vi "slides.vi"() -> ()   [LabVIEW 2020]
uses:
  <instrlib>/_niInstr/Network/IPv4/UDP/Data Stream/v1/niInstr IPv4 UDP Data Stream v1.lvclass
  <instrlib>/_niInstr/Network/IPv4/UDP/Data Stream/v1/Read Data Stream.vi
  <instrlib>/_niInstr/Network/Ethernet/Utility/v1/FPGA/niInstr Ethernet Utilities FPGA v1.lvlib
  <instrlib>/_niInstr/Network/IPv4/FPGA/v1/niInstr IPv4 FPGA v1.lvlib
  <instrlib>/_niInstr/Network/IPv4/UDP/FPGA/v1/niInstr IPv4 UDP FPGA v1.lvlib
  Ethernet MAC - Custom/Ethernet MAC - Custom.lvclass
  <vilib>/rvi/DataTransferAndStorage/Container/XNode/niFpgaContainer.xnode
  <instrlib>/_niInstr/Network/IPv4/UDP/Data Stream/v1/Read End of Good Frame.vi
  <instrlib>/_niInstr/Network/IPv4/UDP/Data Stream/v1/Read End of Bad Frame.vi
  submodules/Market.Data.Common/fpga/my.network.data.stream.ctl
  <vilib>/rvi/FIFO/Fifo_Resource/niFpgaFifoEmulationRefIn.vi
  <instrlib>/_niInstr/Network/Types/v1/MAC Address.ctl
  <instrlib>/_niInstr/Network/Types/v1/niInstr Network Types v1.lvlib
  <instrlib>/_niInstr/Network/Types/v1/IPv4 Address.ctl
  submodules/Market.Data.Common/fpga/orderbook.command.type.ctl
  submodules/Market.Data.Common/fpga/fpganow.common.fpga.lvlib
  submodules/Market.Data.Common/fpga/orderbook.command.ctl
panel:
  out "remaining.qty":u32
  out "seconds":u64
  out "nanoseconds":u64
  out "Add":bool
  out "Edit":bool
  out "Remove":bool
  out "seq no":u32
  out "recv.time":u64
  out "parse.time":u64
  out "canceled.qty":u32
  out "executed.qty":u32
  out "price":u64
  out "symbol":u64
  out "quantity":u32
  out "orderId":u64
  out "side":u8
  out "type":T1
  in  "OrderBook.Command":T2={"type"=enum."AddOrder", "side"=0, "orderId "=0, "quantity"=0, "symbol"=0, "price"=0, "executed.qty"=0, "canceled.qty"=0, "remaining.qty"=0, "seconds"=0, "nanoseconds"=0, "Add"=FALSE, "Edit"=FALSE, "Remove"=FALSE, "seq no"=0, "recv.time"=0, "parse.time"=0}
  in  "Dest Port":u16=8000
  in  "IP Address":T3=[176, 197, 84, 255]
  in  "MAC Address":T4=[176, 197, 84, 255, 244, 135] format="%.0x"
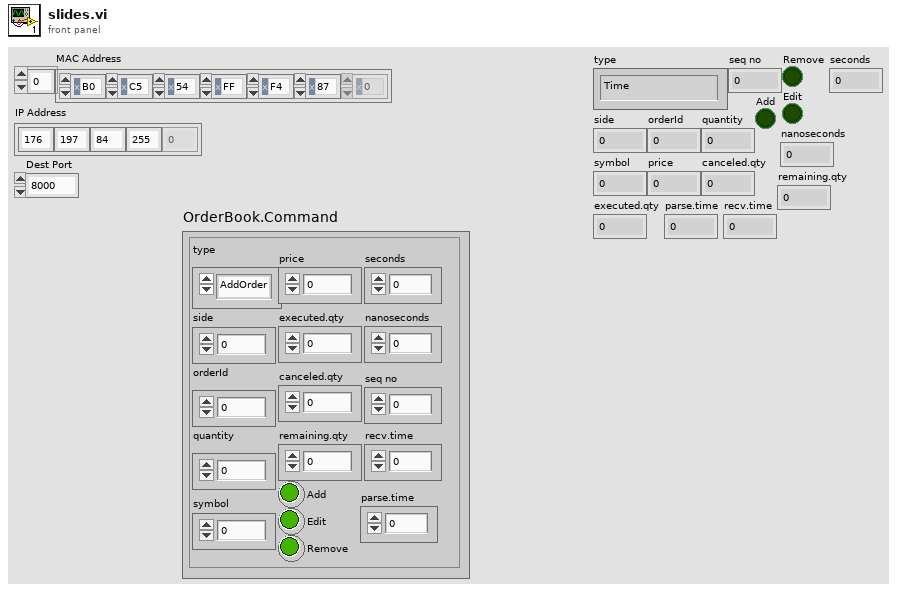
[diagram p1: front panel]
types:
  T1 = typedef "fpganow.common.fpga.lvlib/orderbook.command.type.ctl" = enum8{"Time", "AddOrder", "OrderExecuted", "OrderExecutedAtPrice", "ReduceSize", "ModifyOrder", "DeleteOrder", "Get.Everything", "Get.All.Orders", "Get.Top"}
  T2 = typedef "fpganow.common.fpga.lvlib/orderbook.command.ctl" = cluster{"type":T1, "side":u8, "orderId ":u64, "quantity":u32, "symbol":u64, "price":u64, "executed.qty":u32, "canceled.qty":u32, "remaining.qty":u32, "seconds":u64, "nanoseconds":u64, "Add":bool, "Edit":bool, "Remove":bool, "seq no":u32, "recv.time":u64, "parse.time":u64}
  T3 = typedef "niInstr Network Types v1.lvlib/IPv4 Address.ctl" = u8[]
  T4 = typedef "niInstr Network Types v1.lvlib/MAC Address.ctl" = u8[]
  T5 = typedef "my.network.data.stream.ctl" = cluster{"data":u8[], "data valid":bool, "byte enables":bool[], "eof.good":bool, "eof.bad":bool, "Timestamp":u64}
  T6 = typedef "niInstr Ethernet Utilities FPGA v1.lvlib/Network Data Stream.ctl" = cluster{"data":u8[], "data valid":bool, "byte enables":bool[]}
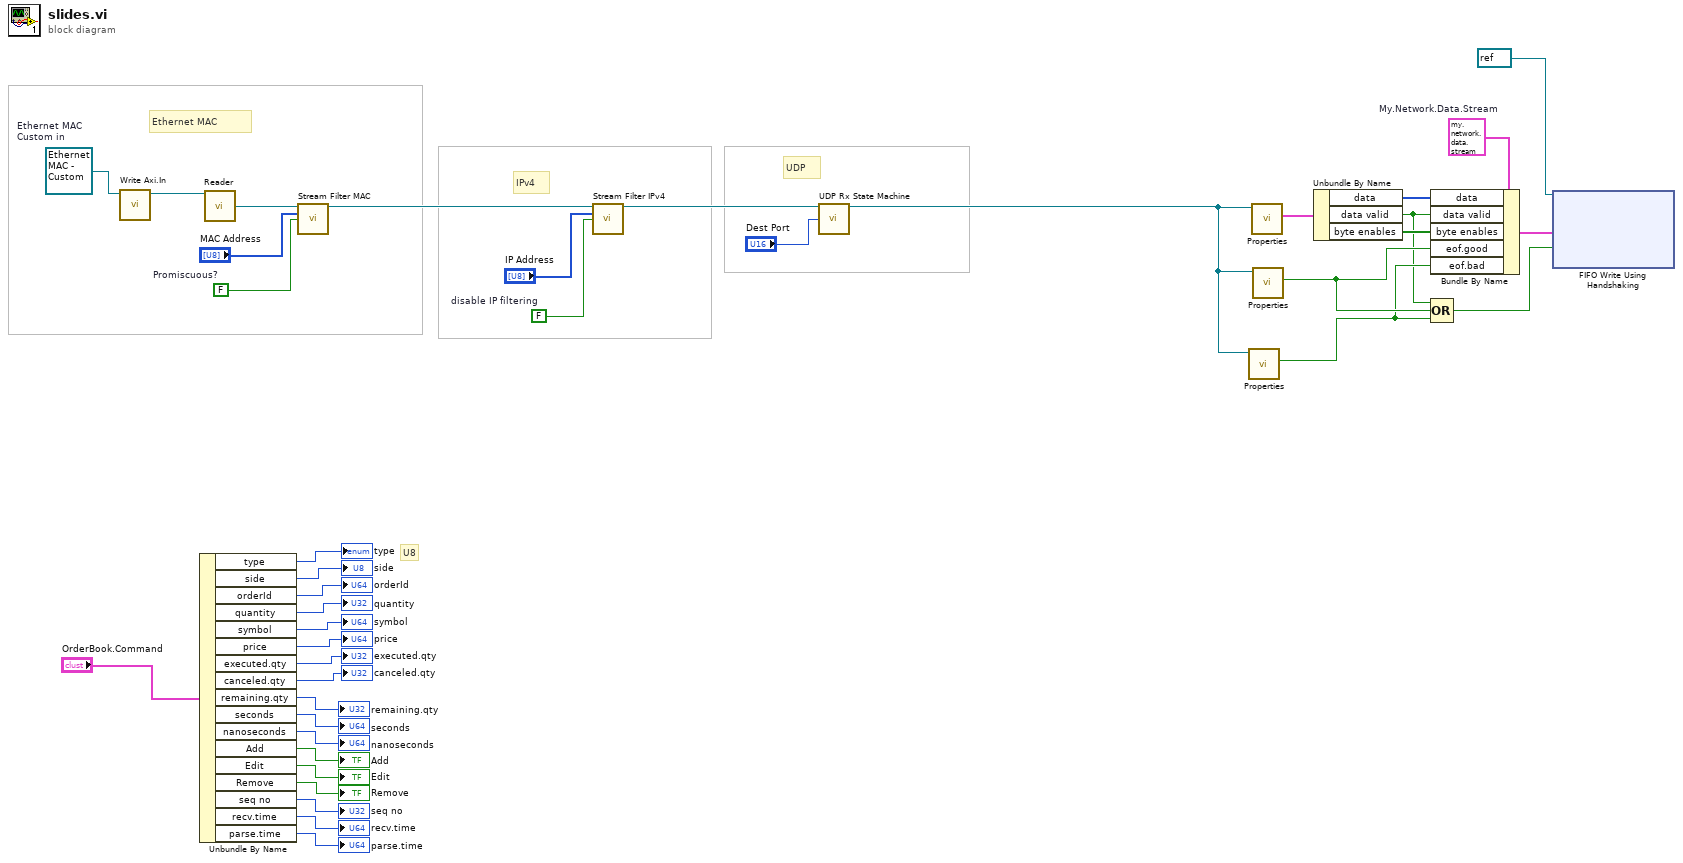
[diagram p0: block diagram]
diagram:
  w29 = T5 {"data"=[0, 0, 0, 0, 0, 0, 0, 0], "data valid"=FALSE, "byte enables"=[FALSE, FALSE, FALSE, FALSE, FALSE, FALSE, FALSE, FALSE], "eof.good"=FALSE, "eof.bad"=FALSE, "Timestamp"=0}  # My.Network.Data.Stream
  w31 = refnum<class "Ethernet MAC - Custom.lvclass"> refnum  # Ethernet MAC Custom in
  w36 = FALSE  # disable IP filtering
  w37 = FALSE  # Promiscuous?
  # "U8"
  # "UDP"
  # "IPv4"
  # "Ethernet MAC"
  n1 = call-dynamic "Write Axi.In.vi"("Ethernet MAC - Custom in"=w31) -> ("Ethernet MAC - Custom out"=w38:refnum<class "Ethernet MAC - Custom.lvclass">)  [unwired: 9 in, 1 out]
  n2 = Unbundle By Name("OrderBook.Command") -> ("type"=→"type":T1, "side"=→"side":u8, "orderId"=→"orderId":u64, "quantity"=→"quantity":u32, "symbol"=→"symbol":u64, "price"=→"price":u64, "executed.qty"=→"executed.qty":u32, "canceled.qty"=→"canceled.qty":u32, "remaining.qty"=→"remaining.qty":u32, "seconds"=→"seconds":u64, "nanoseconds"=→"nanoseconds":u64, "Add"=→"Add":bool, "Edit"=→"Edit":bool, "Remove"=→"Remove":bool, "seq no"=→"seq no":u32, "recv.time"=→"recv.time":u64, "parse.time"=→"parse.time":u64)
  n3 = call-dynamic "Reader.vi"("Ethernet MAC - Custom.lvclass"=w38) -> ("niInstr Ethernet MAC Raw Stream v1.lvclass"=w39:refnum<class "niInstr Ethernet MAC Raw Stream v1.lvclass">)  [unwired: 13 in, 1 out]
  n4 = call <instrlib>:"Stream Filter MAC.vi"("niInstr Ethernet MAC Raw Stream v1 in"=w39, "MAC Address"="MAC Address", "Promiscuous?"=w37) -> ("niInstr Ethernet MAC Data Stream v1 out"=w32:refnum<class "niInstr Ethernet MAC Data Stream v1.lvclass">)  [unwired: 12 in]
  n5 = call <instrlib>:"Stream Filter IPv4.vi"("niInstr Ethernet MAC Data Stream v1 in"=w32, "IP Address"="IP Address", "disable IP filtering"=w36) -> ("niInstr IPv4 Data Stream out"=w20:refnum<class "niInstr IPv4 Data Stream v1.lvclass">)  [unwired: 12 in]
  n6 = call <instrlib>:"UDP Rx State Machine.vi"("niInstr IPv4 Data Stream in"=w20, "Dest Port"="Dest Port") -> ("niInstr IPv4 UDP Data Stream out"=w21:refnum<class "niInstr IPv4 UDP Data Stream v1.lvclass">)  [unwired: 13 in]
  n7 = call-poly <instrlib>:"Properties.vi"("niInstr IPv4 UDP Data Stream in"=w21) -> ("End of Bad Frame"=w24:bool)  [unwired: 9 in, 1 out]
  n8 = call-poly <instrlib>:"Properties.vi"("niInstr IPv4 UDP Data Stream v1.lvclass"=w21) -> ("Data Stream"=w30:T6)  [unwired: 9 in, 1 out]
  n9 = call-poly <instrlib>:"Properties.vi"("niInstr IPv4 UDP Data Stream in"=w21) -> ("End of Good Frame"=w25:bool)  [unwired: 9 in, 1 out]
  n10 = Unbundle By Name(w30) -> ("data"=w23:u8[], "data valid"=w22:bool, "byte enables"=w26:bool[])
  n11 = Bundle By Name(cluster=w29, "data"=w23, "data valid"=w22, "byte enables"=w26, "eof.good"=w25, "eof.bad"=w24) -> (w28:T5)
  n12 = Compound Arithmetic op=OR(w22, w25, w24) -> (w27:bool)
  n13 = xnode "FIFO Write Using Handshaking"("Element"=w28, "Input Valid"=w27, "FIFO In"=refnum<k21> refnum) -> ()  [unwired: 2 out]
